vi "Change Control Labels.vi"(8 "error in (no error)":errorcluster, 11 "vi path":path) -> (0 "error out":errorcluster)   [LabVIEW 2023]
uses:
  <vilib>/Utility/traverseref.llb/VI Scripting - Traverse.lvlib
  <vilib>/Utility/traverseref.llb/TRef TravTarget.ctl
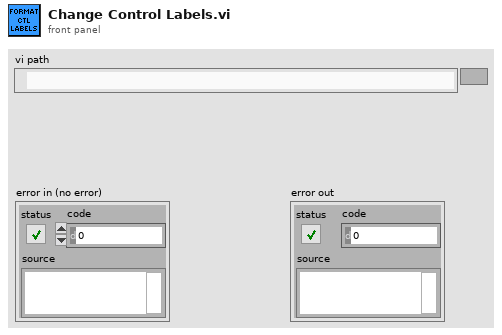
[diagram p1: front panel]
types:
  T1 = typedef "TRef TravTarget.ctl" = enum16{"FP", "BD", "Other"}
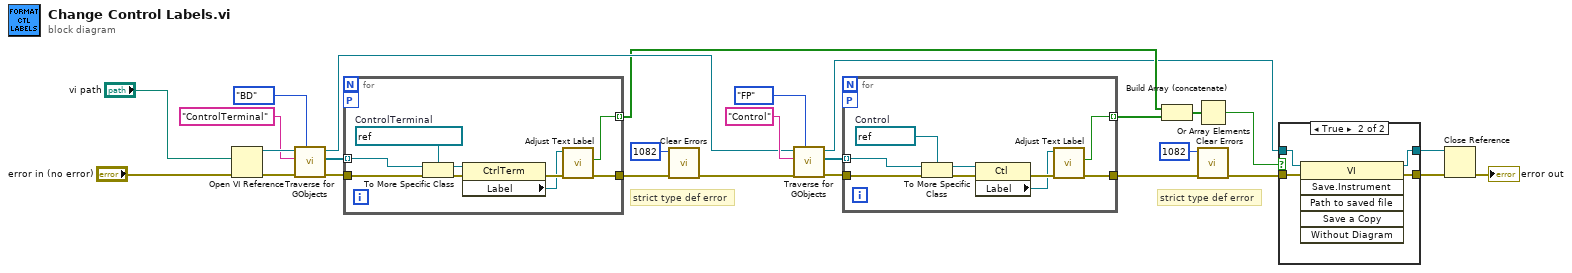
[diagram p0: block diagram]
diagram:
  # "strict type def error"
  # "strict type def error"
  n1 = Open VI Reference(vi path="vi path", error in (no error)="error in (no error)") -> (vi reference=w21:refnum<vi>, error out=w22:errorcluster)  [unwired: 4 in]
  n2 = call <vilib>:"Traverse for GObjects.vi"("Traverse Target"=TRef_TravTarget."BD", "error in (no error)"=w22, "Class Name"="ControlTerminal", "VI Refnum"=w21) -> ("error out"=w19:errorcluster, "References"=w18:refnum<vi>[], "dup VI Refnum"=w12:refnum<vi>)  [unwired: 4 in, 1 out]
  n3 = for {
    tunnel: w18 -> [w36] mode=indexing
    workers-P: _ -> [_]
    tunnel: [w28] -> w10 mode=indexing
    tunnel: w19 -> [w32]
    tunnel: [w30] -> w6
    w35 = refnum<vi> refnum  # ControlTerminal
    n4 = To More Specific Class(target class=w35, reference=w36, error in=w32) -> (specific class reference=w34:refnum<vi>, error out=w33:errorcluster)
    n5 = property class="CtrlTerm"(reference=w34, error in=w33) -> (error out=w31:errorcluster, "Label"=w29:refnum<vi>)  [unwired: 1 out]
    n6 = call "Adjust Text Label.vi"("error in (no error)"=w31, "Label Ref"=w29) -> ("error out"=w30:errorcluster, "Changed?"=w28:bool)  [unwired: 8 in]
  }
  n7 = call <vilib>:"Clear Errors.vi"("error in (no error)"=w6, "specific error code to clear (0: all)"=1082) -> ("error out"=w5:errorcluster)  [unwired: 4 in, 1 out]
  n8 = call <vilib>:"Traverse for GObjects.vi"("Traverse Target"=TRef_TravTarget."FP", "error in (no error)"=w5, "Class Name"="Control", "VI Refnum"=w12) -> ("error out"=w14:errorcluster, "References"=w15:refnum<vi>[], "dup VI Refnum"=w7:refnum<vi>)  [unwired: 4 in, 1 out]
  n9 = for {
    tunnel: w15 -> [w45] mode=indexing
    workers-P: _ -> [_]
    tunnel: [w37] -> w11 mode=indexing
    tunnel: w14 -> [w41]
    tunnel: [w39] -> w2
    w44 = refnum<vi> refnum  # Control
    n10 = To More Specific Class(target class=w44, reference=w45, error in=w41) -> (specific class reference=w43:refnum<vi>, error out=w42:errorcluster)
    n11 = property class="Ctl"(reference=w43, error in=w42) -> (error out=w40:errorcluster, "Label"=w38:refnum<vi>)  [unwired: 1 out]
    n12 = call "Adjust Text Label.vi"("error in (no error)"=w40, "Label Ref"=w38) -> ("error out"=w39:errorcluster, "Changed?"=w37:bool)  [unwired: 8 in]
  }
  n13 = Build Array (concatenate)(w10, w11) -> (w9:bool[])
  n14 = Or Array Elements(Boolean array=w9) -> (logical OR=w8:bool)
  n15 = call <vilib>:"Clear Errors.vi"("error in (no error)"=w2, "specific error code to clear (0: all)"=1082) -> ("error out"=w1:errorcluster)  [unwired: 4 in, 1 out]
  n16 = case shown="True" w8 {
    tunnel: w1 -> [w47 w51]
    tunnel: [w47 w50] -> w24
    tunnel: [w46 w49] -> w23
    tunnel: w7 -> [w46 w48]
    frame False {
    }
    frame True {
      n17 = invoke class="VI" method="Save.Instrument"(reference=w48, error in=w51) -> (reference out=w49:refnum<vi>, error out=w50:errorcluster)  [unwired: 4 in, 4 out]
    }
  }
  n18 = Close Reference(reference=w23, error in (no error)=w24) -> (error out=→"error out":errorcluster)
